vi "梯形面積.vi"() -> ()   [LabVIEW 2019]
uses:
  Control 3.ctl
panel:
  out "Waveform Graph":dbl[](graph)
  in  "Cluster":T1
  out "Waveform Chart":dbl(graph)
  out "Numeric":dbl
  out "Array 3":dbl[](array[numeric])
  in  "Array 2":dbl[][](array[numeric])
  out "element":dbl
  out "size(s)":i32[](array[numeric])
  in  "Array":dbl[][](array[numeric])
  out "x+y":i32
  out "跑的次數":i32
  out "status message":string
  out "warning":bool
  out "時":dbl
  out "分":dbl
  out "秒":dbl
  in  "total seconds":dbl format="%#_13g"
  out "面積":dbl
  in  "下底":dbl
  in  "高":dbl
  in  "上底":dbl
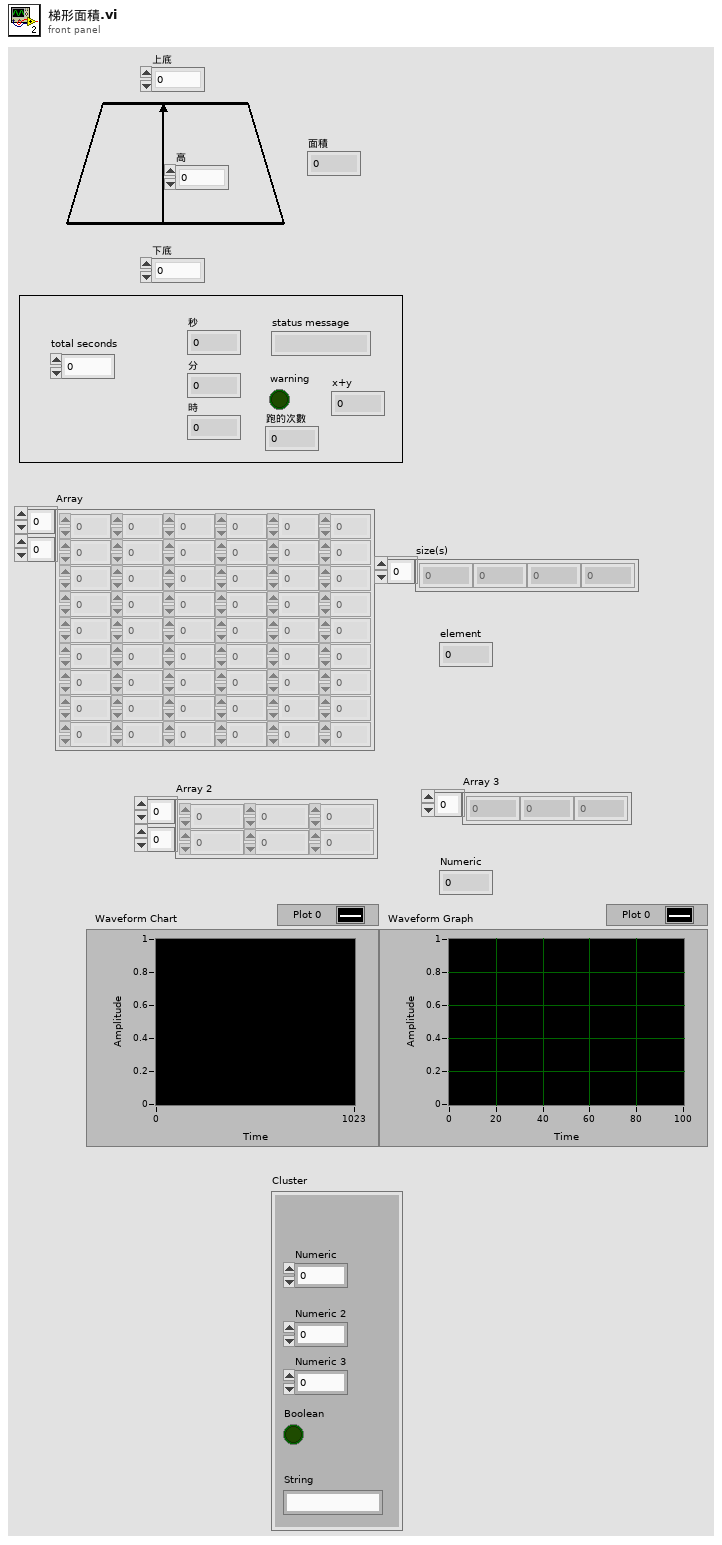
[diagram p1: front panel]
types:
  T1 = cluster{"Numeric":dbl, "Numeric 2":dbl, "Numeric 3":dbl, "Boolean":bool, "String":string}
  T2 = typedef "Control 3.ctl" = enum16{"time check", "data log"}
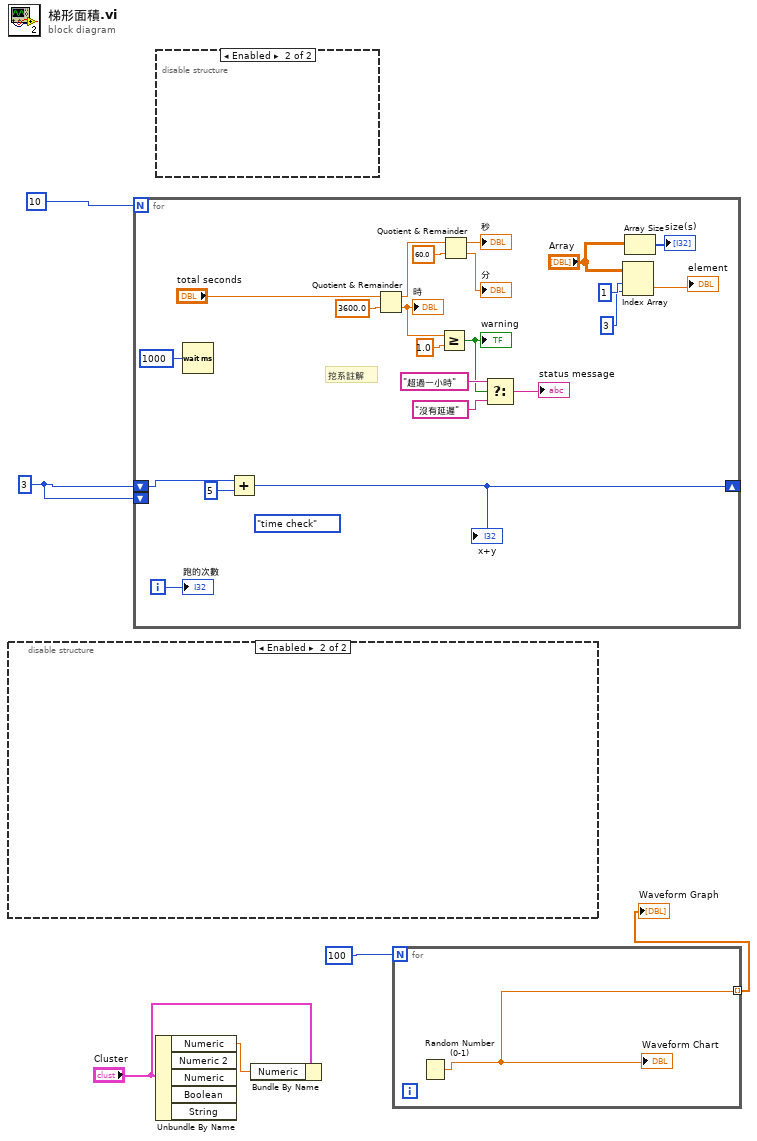
[diagram p0: block diagram]
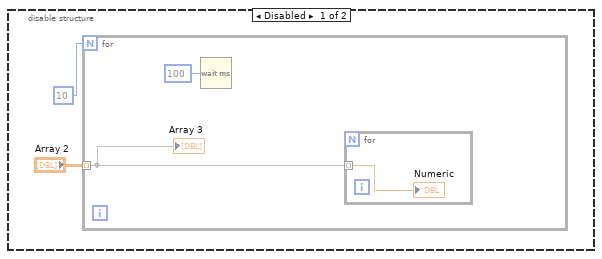
[diagram p2: hidden frame]
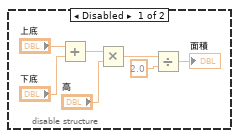
[diagram p3: hidden frame]
diagram:
  w1 = 3
  n1 = disable-structure shown="Enabled" {
    frame Disabled {
      n2 = for {
        N: 10 -> [_]
        tunnel: "Array 2" -> [w10] mode=indexing
        n3 = Wait (ms)(milliseconds to wait=u32 100) -> ()  [unwired: 1 out]
        n4 = for {
          tunnel: w10 -> [w11] mode=indexing
          "Numeric" <- w11
        }
        "Array 3" <- w10
      }
    }
    frame Enabled {
    }
  }
  n5 = for {
    N: 10 -> [_]
    shift-right: [w18] -> _
    shift-left: w1 -> [w19]
    shift-left: w1 -> [_]
    i -> [w21]
    (unwired) Control_3."time check"
    # "挖系註解"
    n6 = Wait (ms)(milliseconds to wait=u32 1000) -> ()  [unwired: 1 out]
    n7 = Add(x=w19, y=5) -> (x+y=w18:i32)
    "x+y" <- w18
    n8 = Quotient & Remainder(x="total seconds", y=3600.0) -> (x-y*floor(x/y)=w31:dbl, floor(x/y)=w27:dbl)
    "時" <- w27
    n9 = Greater Or Equal?(x=w27, y=1.0) -> (x >= y?=w23:bool)
    "warning" <- w23
    n10 = Quotient & Remainder(x=w31, y=60.0) -> (x-y*floor(x/y)=→"秒":dbl, floor(x/y)=→"分":dbl)
    n11 = Select(t="超過一小時", s=w23, f="沒有延遲") -> (s? t:f=→"status message":string)
    n12 = Index Array(array="Array", index (row)=1, index (col)=3 ("disabled index (col)")) -> (element=→"element":dbl)
    n13 = Array Size(array="Array") -> (size(s)=→"size(s)":i32[])
    "跑的次數" <- w21
  }
  n14 = Unbundle By Name("Cluster") -> ("Numeric"=w6:dbl)  [unwired: 4 out]
  n15 = disable-structure shown="Enabled" {
    frame Disabled {
      n16 = Add(x="上底", y="下底") -> (x+y=w38:dbl)
      n17 = Multiply(x=w38, y="高") -> (x*y=w36:dbl)
      n18 = Divide(x=w36, y=2.0) -> (x/y=→"面積":dbl)
    }
    frame Enabled {
    }
  }
  n19 = Bundle By Name(cluster="Cluster", "Numeric"=w6) -> ()  [unwired: 1 out]
  n20 = for {
    N: 100 -> [_]
    tunnel: [w41] -> w3 mode=indexing
    n21 = Random Number (0-1)() -> (number: 0 to 1=w41:dbl)
    "Waveform Chart" <- w41
  }
  "Waveform Graph" <- w3
